vi "密码重置.vi"() -> ()   [LabVIEW 2019]
panel:
  out "错误输出 2":errorcluster caption="错误输出"
  out "error out":errorcluster
  out "用户名：":string
  in  "取消按钮":bool
  in  "新密码：":string
  in  "重复密码：":string
  in  "确定按钮":bool
  # "用户密码修改"
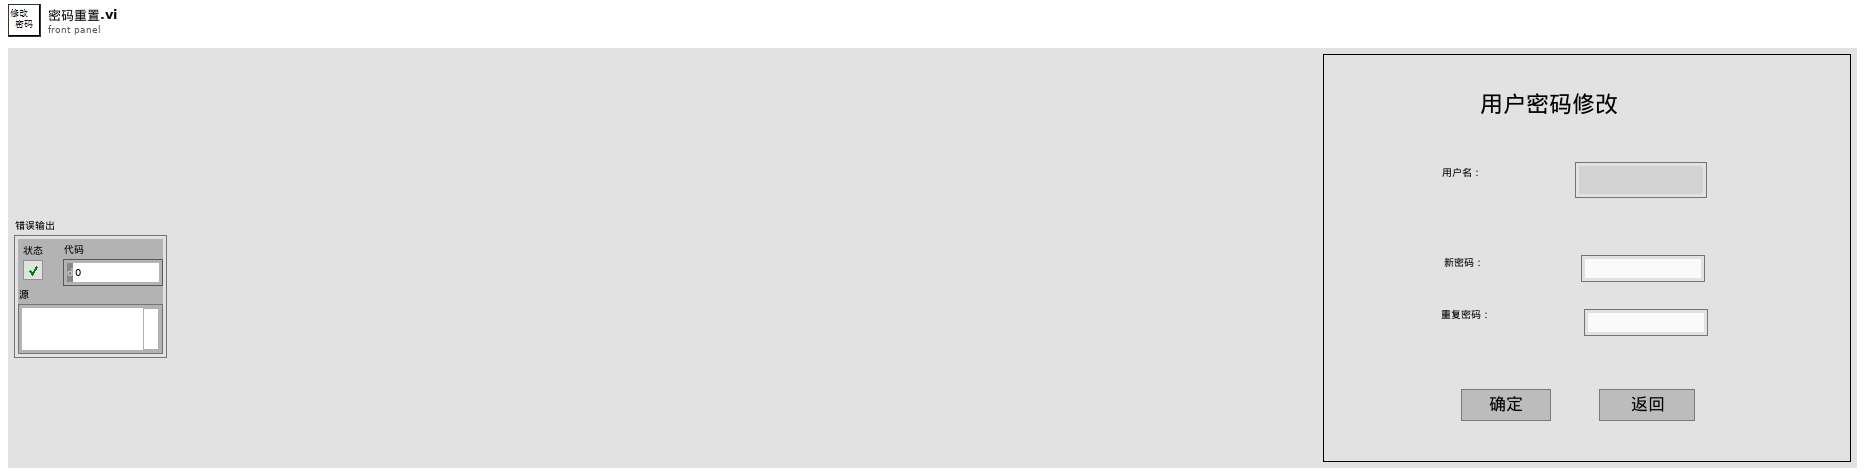
[diagram p1: front panel]
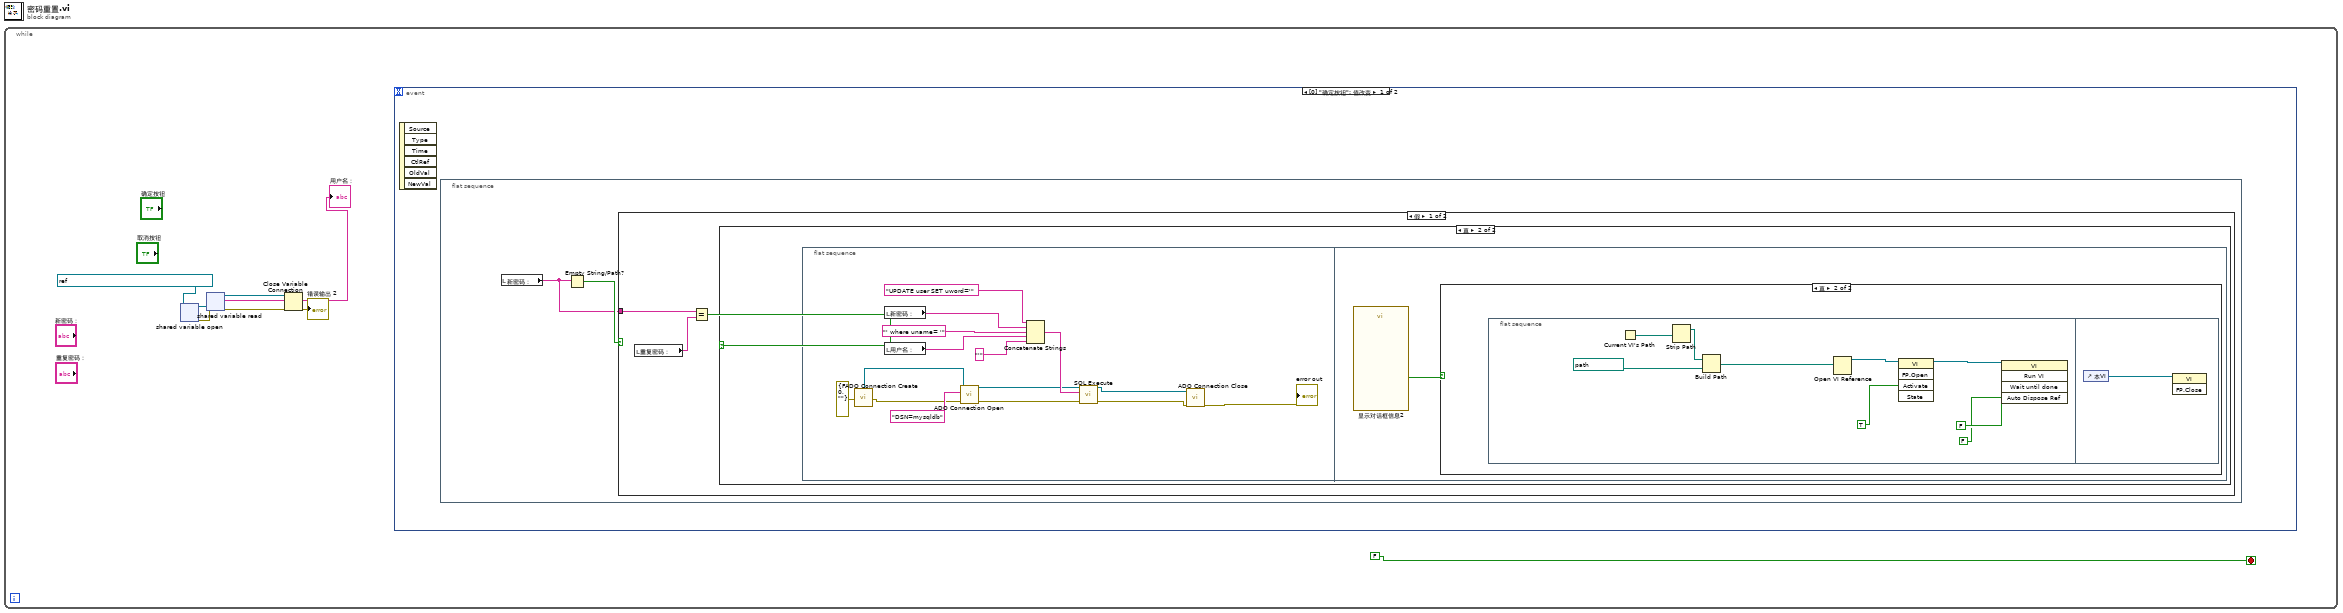
[diagram p0: block diagram]
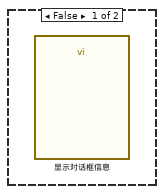
[diagram p2: hidden frame]
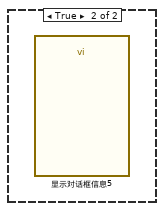
[diagram p4: hidden frame]
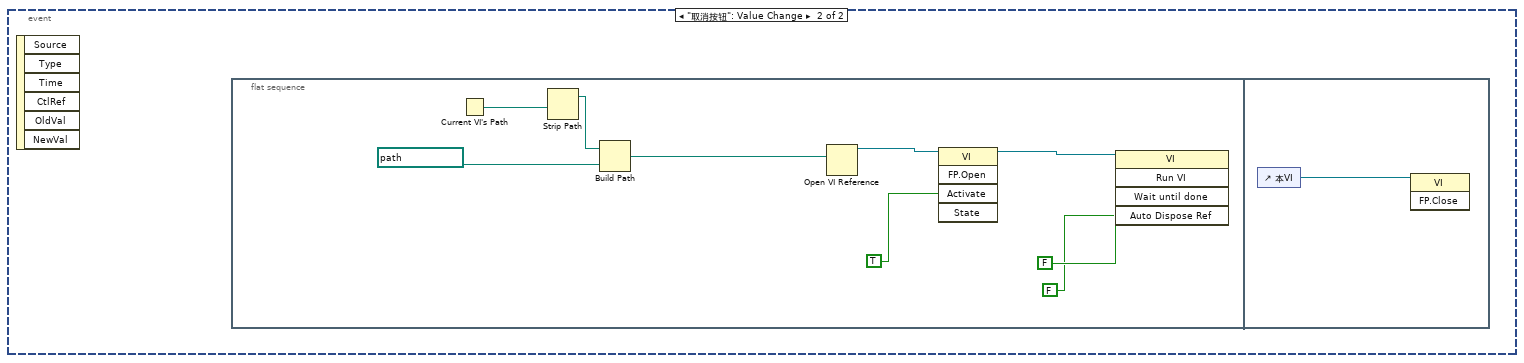
[diagram p5: hidden frame]
diagram:
  n1 = while {
    stop <- FALSE stop-if-true
    n2 = shared-variable-open(refnum<k21> "ni.var.psp://localhost/登录/管理员选择用户" ("共享变量引用句柄输入")) -> (w7:refnum<k21>, w6:errorcluster)  [unwired: 2 in]
    n3 = shared-variable-read(w7, w6) -> (w5:refnum<k21>, w4:errorcluster, →"用户名：":string)  [unwired: 1 out]
    n4 = Close Variable Connection(8:w4, 11:w5) -> (0:→"错误输出 2":errorcluster)
    n5 = event shown="[0] \"确定按钮\": 值改变" {
      selector: _ -> [_ _]
      dyn-events: _ -> [_ _]
      timeout: _ -> [_ _]
      event "确定按钮": Value Change {
        n6 = event-data() -> ()  [unwired: 1 in, 6 out]
        n7 = flat-sequence {
          frame #0 {
            n8 = local read "新密码："() -> (w9:string)
            n9 = Empty String/Path?(string/path=w9) -> (empty?=w10:bool)
            n10 = case shown="假" w10 {
              tunnel: w9 -> [w12 _]
              frame False {
                n11 = local read "重复密码："() -> (w13:string)
                n12 = Equal?(x=w12, y=w13) -> (x = y?=w11:bool)
                n13 = case shown="真" w11 {
                  frame False {
                    n14 = call "显示对话框信息"() -> ()  [unwired: 10 in, 2 out]
                  }
                  frame True {
                    n15 = flat-sequence {
                      frame #0 {
                        n16 = call <userlib>:"ADO Connection Create.vi"("error in (no error)"=errorcluster {"status"=FALSE, "code"=0, "source"=""}) -> ("error out"=w26:errorcluster, "ADODB._Connection Out"=w28:refnum<k7>)  [unwired: 9 in]
                        n17 = local read "新密码："() -> (w22:string)
                        n18 = local read "用户名："() -> (w15:string)
                        n19 = call <userlib>:"ADO Connection Open.vi"("error in (no error)"=w26, "ConnectionString"="DSN=mysqldb", "ADODB._Connection In"=w28) -> ("error out"=w25:errorcluster, "ADODB._Connection Out"=w16:refnum<k7>)  [unwired: 7 in]
                        n20 = Concatenate Strings("UPDATE user SET uword='", w22, "' where uname= '" ("字符串"), w15, "'" ("字符串")) -> (w20:string)
                        n21 = call <userlib>:"SQL Execute.vi"("error in (no error)"=w25, "Command Text"=w20, "ADODB._Connection In"=w16) -> ("error out"=w18:errorcluster, "ADODB._Connection Out"=w17:refnum<k7>)  [unwired: 5 in, 2 out]
                        n22 = call <userlib>:"ADO Connection Close.vi"("error in (no error)"=w18, "ADODB._Connection In"=w17) -> ("error out"=→"error out":errorcluster)  [unwired: 8 in, 1 out]
                      }
                      frame #1 {
                        n23 = call "显示对话框信息2"() -> ("确定"=w29:bool)  [unwired: 10 in, 1 out]
                        n24 = case shown="真" w29 {
                          frame False {
                          }
                          frame True {
                            n25 = flat-sequence {
                              frame #0 {
                                n26 = Current VI's Path() -> (path=w32:path)
                                n27 = Strip Path(path=w32) -> (stripped path=w33:path)  [unwired: 1 out]
                                n28 = Build Path(base path=w33, name or relative path=path "管理员面板.vi") -> (appended path=w31:path)
                                n29 = Open VI Reference(vi path=w31) -> (vi reference=w38:refnum<vi>)  [unwired: 5 in, 1 out]
                                n30 = invoke class="VI" method="FP.Open"(reference=w38, "Activate"=TRUE) -> (reference out=w36:refnum<vi>)  [unwired: 3 in, 4 out]
                                n31 = invoke class="VI" method="Run VI"(reference=w36, "Wait until done"=FALSE, "Auto Dispose Ref"=FALSE) -> ()  [unwired: 2 in, 5 out]
                              }
                              frame #1 {
                                n32 = control-ref of="本VI"() -> (w39:refnum<vi>)
                                n33 = invoke class="VI" method="FP.Close"(reference=w39) -> ()  [unwired: 2 in, 3 out]
                              }
                            }
                          }
                        }
                      }
                    }
                  }
                }
              }
              frame True {
                n34 = call "显示对话框信息5"() -> ()  [unwired: 10 in, 2 out]
              }
            }
          }
        }
      }
      event "取消按钮": Value Change {
        n35 = event-data() -> ()  [unwired: 1 in, 6 out]
        n36 = flat-sequence {
          frame #0 {
            n37 = Current VI's Path() -> (path=w42:path)
            n38 = Strip Path(path=w42) -> (stripped path=w43:path)  [unwired: 1 out]
            n39 = Build Path(base path=w43, name or relative path=path "管理员面板.vi") -> (appended path=w41:path)
            n40 = Open VI Reference(vi path=w41) -> (vi reference=w48:refnum<vi>)  [unwired: 5 in, 1 out]
            n41 = invoke class="VI" method="FP.Open"(reference=w48, "Activate"=TRUE) -> (reference out=w46:refnum<vi>)  [unwired: 3 in, 4 out]
            n42 = invoke class="VI" method="Run VI"(reference=w46, "Wait until done"=FALSE, "Auto Dispose Ref"=FALSE) -> ()  [unwired: 2 in, 5 out]
          }
          frame #1 {
            n43 = control-ref of="本VI"() -> (w49:refnum<vi>)
            n44 = invoke class="VI" method="FP.Close"(reference=w49) -> ()  [unwired: 2 in, 3 out]
          }
        }
      }
    }
  }
